vi "Temperature Warnings.vi"() -> ()   [LabVIEW 2012]
doc: "本VI用于判定基于当前温度值和边界设置的字符串，该字符串输出至气象站。\n\n输入：当前温度值（双精度）、最小温度值（双精度）和最大温度值（双精度）。\n输出：警告文本（字符串）和警告？（布尔）。"
panel:
  out "警告文本":string="无警告"
  out "警告？":bool
  in  "最低温度":dbl
  in  "最高温度":dbl
  in  "当前温度":dbl
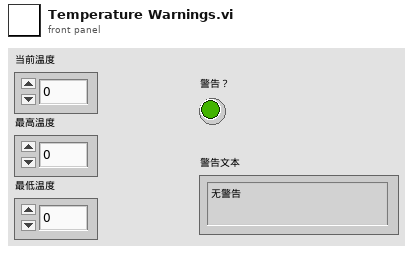
[diagram p1: front panel]
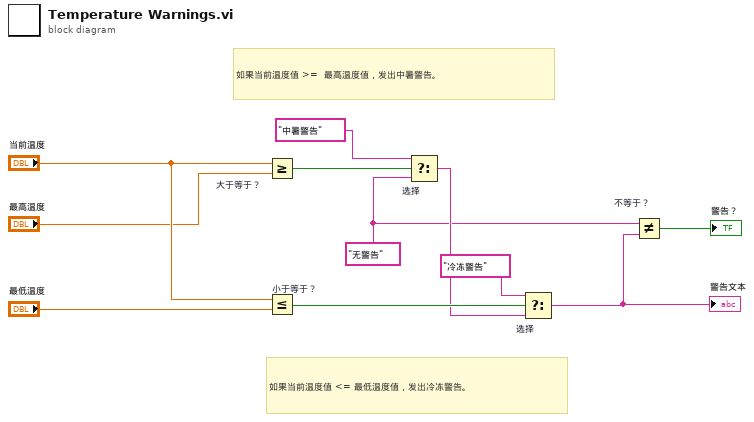
[diagram p0: block diagram]
diagram:
  w1 = "无警告" ("f")
  # "如果当前温度值 >=  最高温度值，发出中暑警告。"
  # "如果当前温度值 <= 最低温度值，发出冷冻警告。"
  n1 = Greater Or Equal? "大于等于？"(x="当前温度", y="最高温度") -> (x >= y?=w6:bool)
  n2 = Less Or Equal? "小于等于？"(x="当前温度", y="最低温度") -> (x <= y?=w3:bool)
  n3 = Select "选择"(t="中暑警告", s=w6, f=w1) -> (s? t:f=w2:string)
  n4 = Select "选择"(t="冷冻警告", s=w3, f=w2) -> (s? t:f=w7:string)
  "警告文本" <- w7
  n5 = Not Equal? "不等于？"(x=w1, y=w7) -> (x != y?=→"警告？":bool)
